vi "NI DAQ globals.vi"() -> ()   [LabVIEW 2020]
panel:
  out "trigger task":refnum<k21>
  out "clock ref 5 MHz task":refnum<k21>
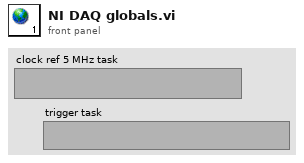
[diagram p1: front panel]
diagram:
